vi "Read.vi"(0 "CS in":refnum<class "CS.lvclass">, 5 "error in (no error)":errorcluster, 6 "Optional":bool) -> (14 "CS out":refnum<class "CS.lvclass">, 15 "I0":T1 {"Current" min=0.0}, 16 "I1":T1 {"Current" min=0.0}, 17 "I2":T1 {"Current" min=0.0}, 18 "I3":T1 {"Current" min=0.0}, 19 "error out":errorcluster)   [LabVIEW 2013, in "CS.lvclass"]
uses:
  Lib.llb/CS.lvclass
  Lib.llb/CS Data.ctl
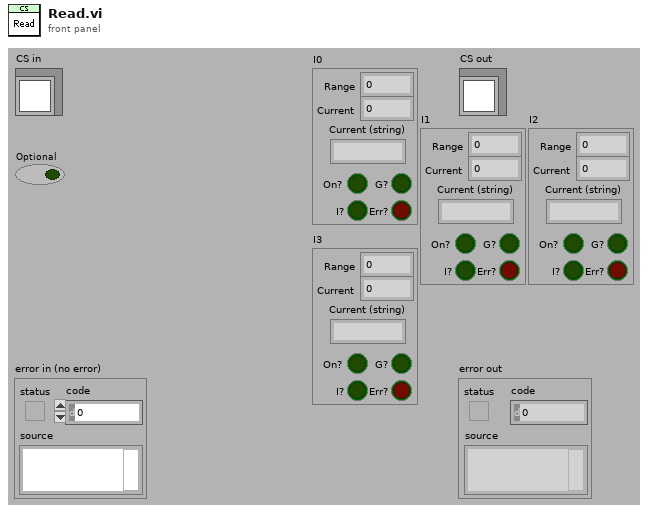
[diagram p1: front panel]
types:
  T1 = typedef "CS Data.ctl" = cluster{"Range":u8, "Current":dbl, "Current (string)":string, "On?":bool, "G?":bool, "I?":bool, "Err?":bool}
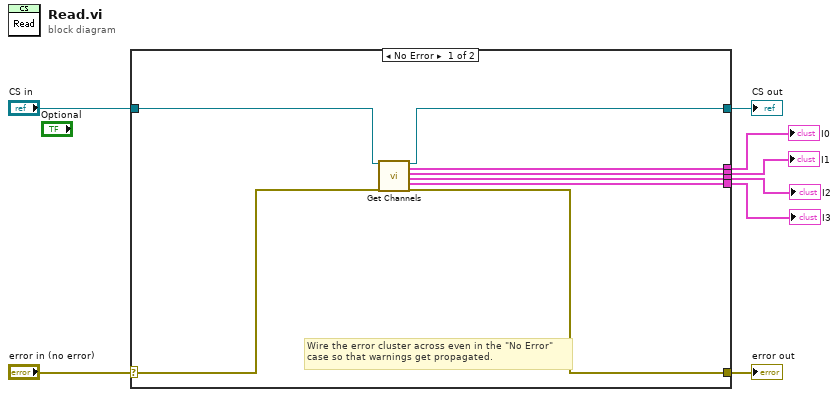
[diagram p0: block diagram]
diagram:
  n1 = case shown="No Error" "error in (no error)" {
    selector: "error in (no error)" -> [w14 w18]
    tunnel: [w13 w18] -> w7
    tunnel: [w15 w17] -> w5
    tunnel: "CS in" -> [w16 w17]
    tunnel: [w12 _] -> w4
    tunnel: [w11 _] -> w3
    tunnel: [w10 _] -> w2
    tunnel: [w9 _] -> w1
    frame No Error {
      # "Wire the error cluster across even in the \"No Error\"\ncase so that warnings get propagated."
      n2 = call-dynamic "Get Channels.vi"("CS.lvclass in"=w16, "error in (no error)"=w14) -> ("CS.lvclass out"=w15:refnum<class "CS.lvclass">, "I0"=w12:T1, "I1"=w11:T1, "I2"=w10:T1, "I3"=w9:T1, "error out"=w13:errorcluster)  [unwired: 12 in]
    }
    frame Error {
    }
  }
  "error out" <- w7
  "CS out" <- w5
  "I0" <- w4
  "I1" <- w3
  "I2" <- w2
  "I3" <- w1
